vi "Parse Message.vi"(8 "error in (no error)":errorcluster, 10 "Data":string, 11 "OBS in":refnum<class "OBS.lvclass">) -> (0 "error out":errorcluster, 2 "Server Message":refnum<class "Server Message.lvclass">, 3 "OBS out":refnum<class "OBS.lvclass">)   [LabVIEW 2020, in "obs-websocket.lvlib" / "OBS.lvclass"]
uses:
  OBS.lvclass
  Server Message/Server Message.lvclass
  Hello/Hello.lvclass
  C:/dev/lv20CE/relink/lv-obs-websocket/obs-websocket/Server Message/Server Message.lvclass
  Identified/Identified.lvclass
  Event/Event.lvclass
  Response/Response.lvclass
  BatchResponse/BatchResponse.lvclass
  c80a257d-e868-4c8c-a4be-f675f36646db.vi
  <vilib>/JDP Science/JSONtext/Next JSON Value.vi
  <vilib>/JDP Science/JSONtext/String Subset.vi
  <vilib>/JDP Science/JSONtext/Parsing/Advance past next JSON Value (inlined COPY).vi
  <vilib>/JDP Science/JSONtext/Parsing/Advance past whitespace.vi
  <vilib>/JDP Science/JSONtext/Parsing/Advance past String.vi
  <vilib>/JDP Science/JSONtext/Parsing/Advance past Number.vi
  <vilib>/JDP Science/JSONtext/Parsing/Advance past Line Ending.vi
  <vilib>/JDP Science/JSONtext/Parsing/Parse Full Path or Item Name.vi
  <vilib>/JDP Science/JSONtext/Parsing/Advance past Array.vi
  <vilib>/JDP Science/JSONtext/Parsing/Advance past Object.vi
  <vilib>/JDP Science/JSONtext/support/Error Cluster From Code.vi
  <vilib>/JDP Science/JSONtext/Offset/Find Item Locations by Path.vi
  <vilib>/JDP Science/JSONtext/JSON text to Variant.vi
  <vilib>/JDP Science/JSONtext/LVClass Serializer/JSONtext LVClass Serializer.lvclass
  obs-websocket.lvlib
  <vilib>/JDP Science/JSONtext/JSONtext.lvlib
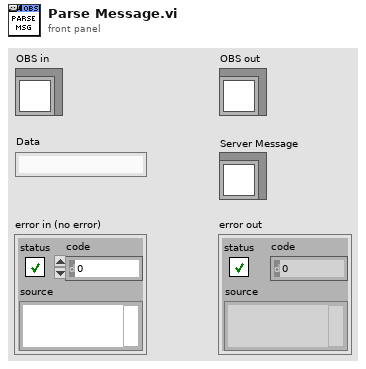
[diagram p1: front panel]
types:
  T1 = typedef "obs-websocket.lvlib/Server Operation.ctl" = enum16{"Hello", "Identified", "Event", "RequestResponse", "RequestBatchResponse"}
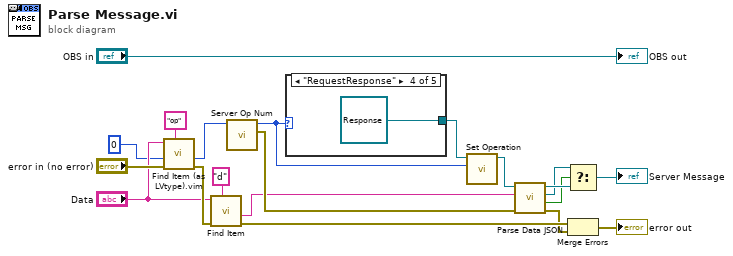
[diagram p0: block diagram]
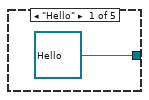
[diagram p2: hidden frame]
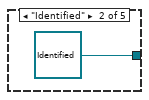
[diagram p3: hidden frame]
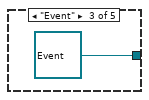
[diagram p4: hidden frame]
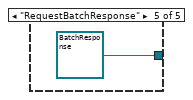
[diagram p5: hidden frame]
diagram:
  n1 = call "Find Item (as LVtype).vim"("$Path or Item Name"="op", "error in (no error)"="error in (no error)", "Data Type and Default Value"=0, "JSON"="Data") -> ("error out"=w18:errorcluster, "Data"=w2:i32)  [unwired: 4 in, 2 out]
  n2 = call <vilib>:"Find Item.vi"("$Path or Item Name"="d", "error in (no error)"=w18, "JSON"="Data") -> ("error out"=w20:errorcluster, "<JSON>"=w1:string)  [unwired: 5 in, 2 out]
  n3 = call "Server Op Num.vi"("Server Op Num"=w2) -> ("error out"=w14:errorcluster, "Server Operation"=w11:T1)  [unwired: 9 in]
  n4 = case shown="\"RequestResponse\"" w11 {
    tunnel: [refnum<class "Hello.lvclass"> refnum ("obs-websocket-lv.lvlib:Hello.lvclass") refnum<class "Identified.lvclass"> refnum ("obs-websocket-lv.lvlib:Identified.lvclass") refnum<class "Event.lvclass"> refnum ("obs-websocket-lv.lvlib:Event.lvclass") refnum<class "Response.lvclass"> refnum ("obs-websocket-lv.lvlib:Response.lvclass") refnum<class "BatchResponse.lvclass"> refnum ("obs-websocket-lv.lvlib:BatchResponse.lvclass")] -> w12
    frame "Hello" {
    }
    frame "Identified" {
    }
    frame "Event" {
    }
    frame "RequestResponse" {
    }
    frame "RequestBatchResponse" {
    }
  }
  n5 = call "Set Operation.vi"("Server Operation"=w11, "Server Message in"=w12) -> ("Server Message out"=w13:refnum<class "Server Message.lvclass">)  [unwired: 8 in, 1 out]
  n6 = call-dynamic "Parse Data JSON.vi"("error in (no error)"=w14, "Data JSON"=w1, "Server Message in"=w13) -> ("error out"=w15:errorcluster, "Replaced?"=w8:bool, "Typed Message"=w9:refnum<class "Response.lvclass">, "Server Message out"=w10:refnum<class "Server Message.lvclass">)  [unwired: 5 in]
  n7 = Select(t=w9, s=w8, f=w10) -> (s? t:f=→"Server Message":refnum<class "Server Message.lvclass">)
  n8 = Merge Errors(w20, w15) -> (→"error out":errorcluster)
  "OBS out" <- "OBS in"
